vi "Pre Launch Init.vi"(11 "IED in":refnum<class "IED.lvclass">) -> (0 "error out":errorcluster, 3 "IED out":refnum<class "IED.lvclass">)   [LabVIEW 2018, in "IED Actor.lvlib" / "IED.lvclass"]
doc: "(<B>Filename</B>: Actor Framework.lvlib:Actor.lvclass:Pre Launch Init.vi)\n\nDefines behavior that occurs after the Launch Nested Actor method is invoked but before the actor's Actor Core method begins running.\n\nBy default, this method does nothing. A descendant class may override it to define behavior."
uses:
  IED.lvclass
  C:/Users/Administrator/Desktop/2018LabVIEW EMS/EMS Generic Actor/EMS Generic/EMS Generic.lvclass
  C:/Users/Administrator/Desktop/2018LabVIEW EMS/IED Actors/Device DDS Communications Framework/Device DDS Communications/Device DDS Communications.lvclass
  IED.lvclass/IED.ctl
  Device DDS Communications Framework/Device DDS Communications/Device DDS Communications.lvclass/Device DDS Communications.ctl
  <vilib>/ORNL/CSEISMIC DDS/CSEISMIC DDS Base/CSEISMIC DDS.lvclass/CSEISMIC DDS.ctl
  <vilib>/ORNL/CSEISMIC DDS/CSEISMIC DDS Base/Accessors/Write DDS Reference.vi
  <vilib>/ORNL/CSEISMIC DDS/DDS Writer/DDS Writer.lvclass
  C:/Program Files (x86)/National Instruments/LabVIEW 2018/vi.lib/ORNL/CSEISMIC DDS/CSEISMIC DDS Base/CSEISMIC DDS.lvclass
  <vilib>/ORNL/CSEISMIC DDS/CSEISMIC DDS Base/Error Handler.vi
  Device DDS Communications Framework/Device DDS Communications/Device DDS Communications.lvclass
  EMS Generic Actor/EMS Generic/EMS Generic.lvclass
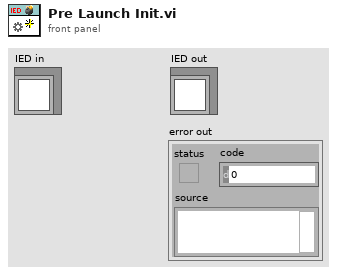
[diagram p1: front panel]
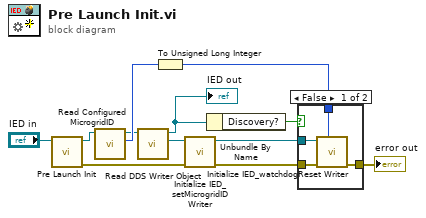
[diagram p0: block diagram]
diagram:
  n1 = call-parent "Pre Launch Init.vi"("Device DDS Communications in"="IED in") -> ("error out"=w7:errorcluster, "Device DDS Communications out"=w5:refnum<class "IED.lvclass">)  [unwired: 9 in]
  n2 = call "Read Configured MicrogridID.vi"("EMS Generic in"=w5) -> ("Microgrid ID"=w10:u8, "EMS Generic out"=w4:refnum<class "IED.lvclass">)  [unwired: 8 in, 1 out]
  n3 = call "Read DDS Writer Object.vi"("Device DDS Communications in"=w4) -> ("DDS Writer Object"=w12:refnum<class "DDS Writer.lvclass">, "Device DDS Communications out"=w2:refnum<class "IED.lvclass">)  [unwired: 9 in]
  "IED out" <- w2
  n4 = To Unsigned Long Integer(number=w10) -> (unsigned 32bit integer=w3:u32)
  n5 = call <vilib>:"Initialize IED_setMicrogridID Writer.vi"("error in"=w7, "DDS Writer in"=w12) -> ("error out"=w9:errorcluster, "DDS Writer out"=w11:refnum<class "DDS Writer.lvclass">)  [unwired: 8 in]
  n6 = Unbundle By Name(w2) -> ("Discovery?"=w1:bool)
  n7 = case shown="False" w1 {
    tunnel: w11 -> [w16 _]
    tunnel: w9 -> [w15 w17]
    tunnel: [w14 w17] -> w8
    tunnel: w3 -> [w13 _]
    frame False {
      n8 = call <vilib>:"Initialize IED_watchdogReset Writer.vi"("MicrogridID"=w13, "error in"=w15, "DDS Writer in"=w16) -> ("error out"=w14:errorcluster)  [unwired: 7 in, 1 out]
    }
    frame True {
    }
  }
  "error out" <- w8
